vi "Const frame i keyword.vi"() -> (2 "Const frame i keyword 2":string[](array[string]), 3 "Const frame i keyword":string[](array[string]))   [LabVIEW 2018, in "Frame Analizer.lvclass"]
uses:
  Frame Analizer.lvclass
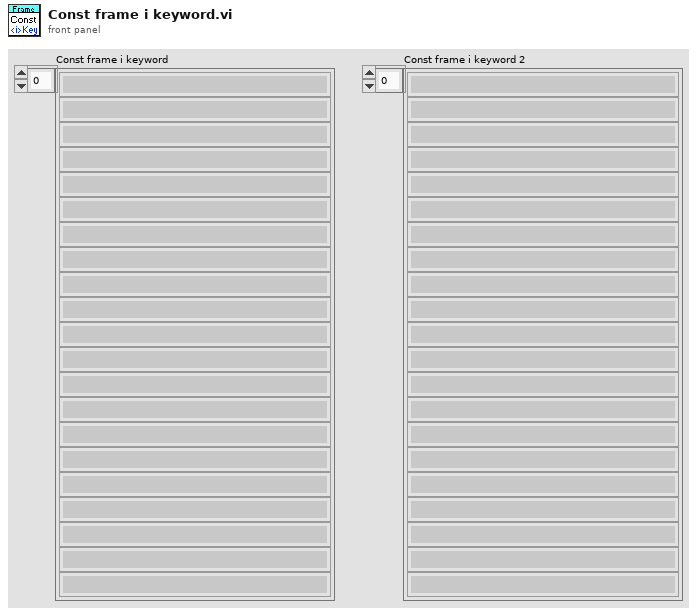
[diagram p1: front panel]
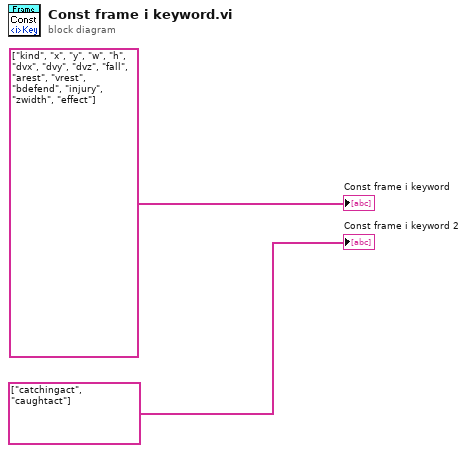
[diagram p0: block diagram]
diagram:
  "Const frame i keyword" <- string[] ["kind", "x", "y", "w", "h", "dvx", "dvy", "dvz", "fall", "arest", "vrest", "bdefend", "injury", "zwidth", "effect"]
  "Const frame i keyword 2" <- string[] ["catchingact", "caughtact"]
